vi "util_Change Detector.vi"(1 "value":variant) -> (0 "changed?":bool)   [LabVIEW 2017]
doc: "Version 3.0, Mar 2001, David A. Moore\nReport if input has changed since previous call. Always false on first call.\n\n3.0: Replaced polymorphic input with Variant input.\n2.0: Added first call logic.\n1.0: From \"Changing Values\" by Meg F. Kay in LabVIEW Technical Resource Volume 4 Number 1."
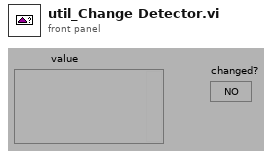
[diagram p1: front panel]
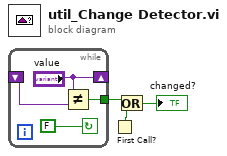
[diagram p0: block diagram]
diagram:
  n1 = while {
    tunnel: [w5] -> w3
    shift-left: _ -> [w7]
    shift-right: ["value"] -> _
    stop <- FALSE continue-if-true
    n2 = Not Equal?(x="value", y=w7) -> (x != y?=w5:bool)
  }
  n3 = First Call?() -> (First Call?: T/F=w2:bool)
  n4 = Or(x=w3, y=w2) -> (x .or. y?=→"changed?":bool)
